vi "Measurement.UI.SetControllerDependency.vi"(8 "error in (no error)":errorcluster, 10 "Measurement":refnum<class "Measurement.lvclass">, 11 "Measurement.UI in":refnum<class "Measurement.UI.lvclass">) -> (0 "error out":errorcluster, 3 "Measurement.UI out":refnum<class "Measurement.UI.lvclass">)   [LabVIEW 2017, in "Measurement.UI.lvclass"]
uses:
  Measurement.UI.lvclass
  Measurement/Measurement.lvclass
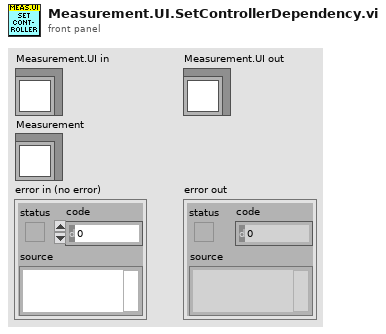
[diagram p1: front panel]
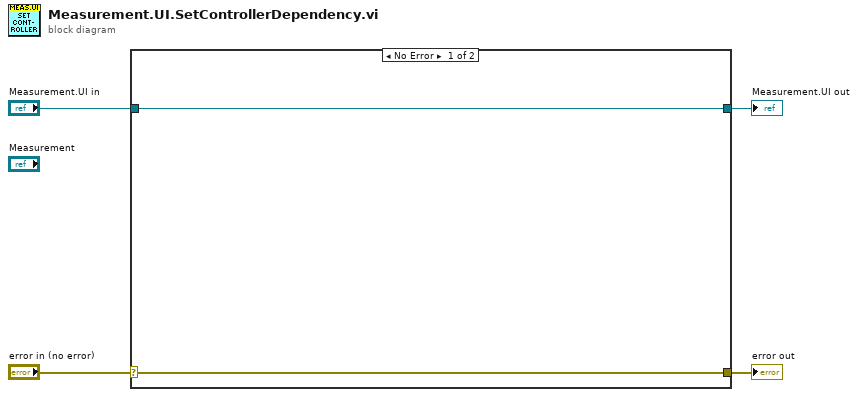
[diagram p0: block diagram]
diagram:
  n1 = case shown="No Error" "error in (no error)" {
    selector: "error in (no error)" -> [w5 w8]
    tunnel: [w5 w8] -> w3
    tunnel: [w6 w7] -> w1
    tunnel: "Measurement.UI in" -> [w6 w7]
    frame No Error {
    }
    frame Error {
    }
  }
  "error out" <- w3
  "Measurement.UI out" <- w1
